vi "Get CameraTimestampTicks and Lostpackages.vi"(8 "error in (no error)":errorcluster, 11 "image in":T1) -> (0 "error out":errorcluster, 1 "Lost Packages":i32, 2 "CameraTimestampTicks":u64, 3 "image dup":T1)   [LabVIEW 2020, in "IMAQdx Actor.lvlib" / "IMAQdx Actor.lvclass"]
uses:
  IMAQdx Actor.lvclass
  <vilib>/vision/Image Controls.llb/IMAQ Image.ctl
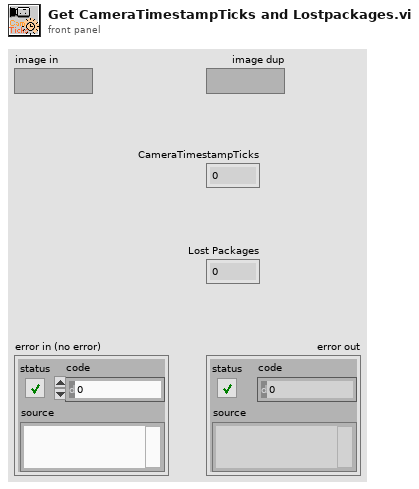
[diagram p1: front panel]
types:
  T1 = typedef "IMAQ Image.ctl" = refnum<image>
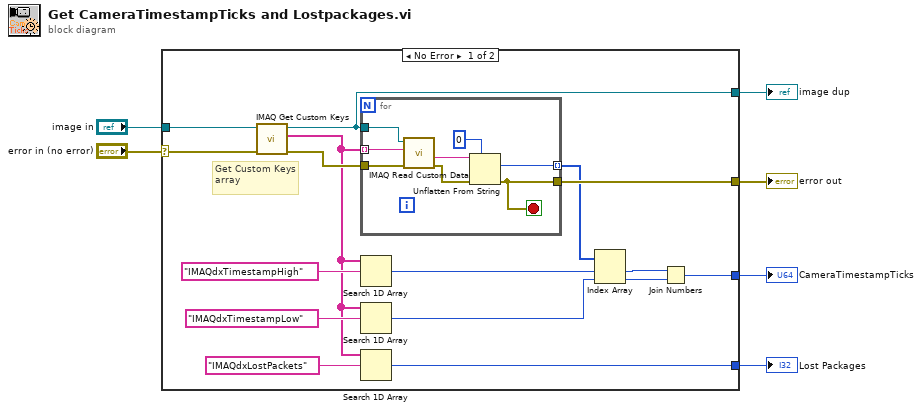
[diagram p0: block diagram]
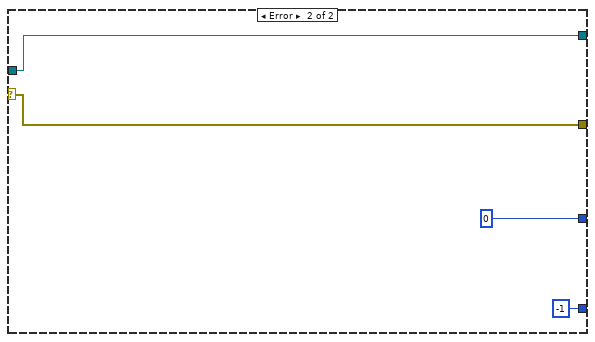
[diagram p2: hidden frame]
diagram:
  n1 = case shown="No Error" "error in (no error)" {
    selector: "error in (no error)" -> [w21 w33]
    tunnel: [w22 w34] -> w6
    tunnel: [w20 w33] -> w4
    tunnel: "image in" -> [w19 w34]
    tunnel: [w10 u64 0] -> w2
    tunnel: [w7 -1 ("index of element")] -> w1
    frame No Error {
      # "Get Custom Keys array"
      n2 = call "IMAQ Get Custom Keys"("error in (no error)"=w21, "Image"=w19) -> ("error out"=w18:errorcluster, "Keys"=w8:string[], "Image (duplicate)"=w22:T1)  [unwired: 6 in, 1 out]
      n3 = for {
        tunnel: w22 -> [w30]
        tunnel: w18 -> [w29]
        tunnel: [w23] -> w20
        tunnel: w8 -> [w28] mode=indexing
        tunnel: [w27] -> w17 mode=indexing
        stop <- w23 stop-if-true
        n4 = call "IMAQ Read Custom Data"("error in (no error)"=w29, "Key"=w28, "Image"=w30) -> ("error out"=w26:errorcluster, "Custom Data Out"=w25:string)  [unwired: 6 in, 1 out]
        n5 = Unflatten From String(type=0, binary string=w25, error in (no error)=w26) -> (value=w27:i32, error out=w23:errorcluster)  [unwired: 2 in, 1 out]
      }
      n6 = Search 1D Array(1D array=w8, element="IMAQdxTimestampHigh") -> (index of element=w13:i32)  [unwired: 1 in]
      n7 = Search 1D Array(1D array=w8, element="IMAQdxTimestampLow") -> (index of element=w14:i32)  [unwired: 1 in]
      n8 = Search 1D Array(1D array=w8, element="IMAQdxLostPackets") -> (index of element=w7:i32)  [unwired: 1 in]
      n9 = Index Array(array=w17, index #1=w13, index #2=w14) -> (element #1=w11:i32, element #2=w12:i32)
      n10 = Join Numbers(hi=w11, lo=w12) -> ((hi.lo)=w10:u64)
    }
    frame Error {
    }
  }
  "image dup" <- w6
  "error out" <- w4
  "CameraTimestampTicks" <- w2
  "Lost Packages" <- w1
